vi "Calibration GUI.vi"(7 "Actions":T1, 8 "error in (no error)":errorcluster, 10 "index":i32, 11 "Ctrl Ref":refnum<vi>[](array[refnum])) -> (0 "error out":errorcluster)   [LabVIEW 2011]
uses:
  Controls/typedef_enum_GFV Calibration GUI_actions.ctl
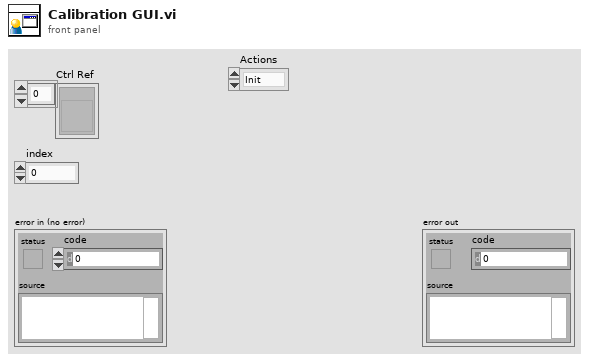
[diagram p1: front panel]
types:
  T1 = typedef "typedef_enum_GFV Calibration GUI_actions.ctl" = enum16{"Init", "Update GUI", "Clear GUI"}
  T2 = enum8{"Enabled", "Disabled", "Disabled and Grayed Out"}
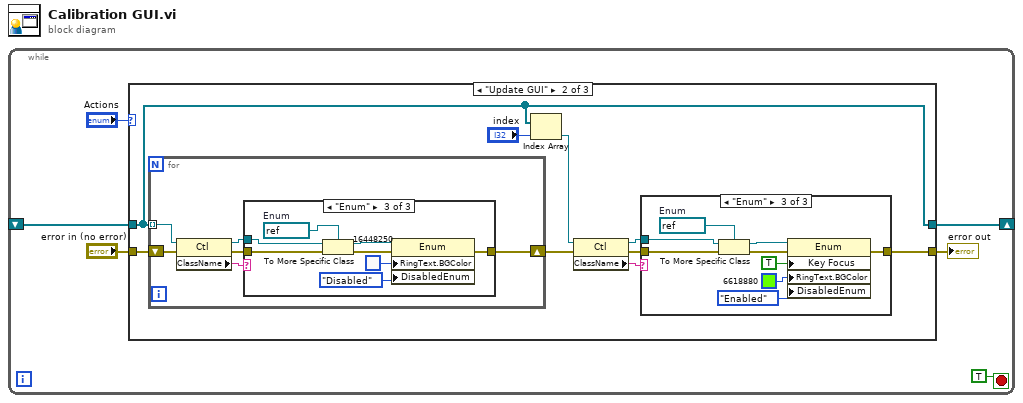
[diagram p0: block diagram]
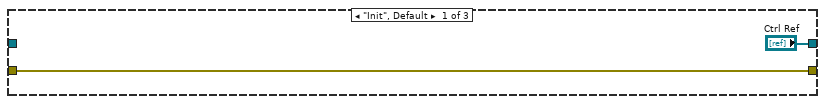
[diagram p2: hidden frame]
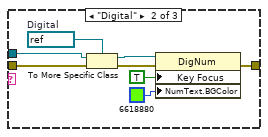
[diagram p4: hidden frame]
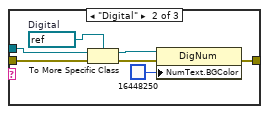
[diagram p6: hidden frame]
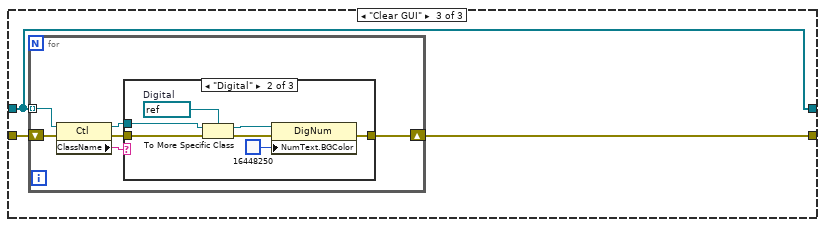
[diagram p7: hidden frame]
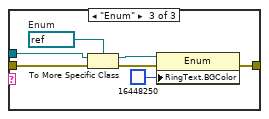
[diagram p9: hidden frame]
diagram:
  n1 = while {
    shift-right: [w2] -> _
    shift-left: _ -> [w1]
    stop <- TRUE stop-if-true
    n2 = case shown="\"Update GUI\"" "Actions" {
      tunnel: [w7 w10 w58] -> w6
      tunnel: "error in (no error)" -> [w7 w17 w60]
      tunnel: ["Ctrl Ref" w15 w59] -> w2
      tunnel: w1 -> [_ w15 w59]
      frame "Init", Default {
      }
      frame "Update GUI" {
        n3 = for {
          tunnel: w15 -> [w41] mode=indexing
          shift-right: [w36] -> w9
          shift-left: w17 -> [w37]
          n4 = property on="Property Node" class="Ctl"(reference=w41, error in=w37) -> (reference out=w39:refnum<vi>, error out=w38:errorcluster, "ClassName"=w40:string)
          n5 = case shown="\"Enum\"" w40 {
            tunnel: w39 -> [_ w47 w55]
            tunnel: w38 -> [w42 w46 w54]
            tunnel: [w42 w45 w53] -> w36
            frame "False", Default {
            }
            frame "Digital" {
              w43 = refnum<vi> refnum  # Digital
              n6 = To More Specific Class(target class=w43, reference=w47, error in=w46) -> (specific class reference=w44:refnum<vi>, error out=w48:errorcluster)
              n7 = property on="Property Node" class="DigNum"(reference=w44, error in=w48, "NumText.BGColor"=u32 16448250) -> (error out=w45:errorcluster)  [unwired: 1 out]
            }
            frame "Enum" {
              w51 = refnum<vi> refnum  # Enum
              n8 = To More Specific Class(target class=w51, reference=w55, error in=w54) -> (specific class reference=w52:refnum<vi>, error out=w56:errorcluster)
              n9 = property on="Property Node" class="Enum"(reference=w52, error in=w56, "RingText.BGColor"=u32 16448250, "DisabledEnum"=T2."Disabled" ("Disabled")) -> (error out=w53:errorcluster)  [unwired: 1 out]
            }
          }
        }
        n10 = Index Array(array=w15, index="index") -> (element=w11:refnum<vi>)
        n11 = property on="Property Node" class="Ctl"(reference=w11, error in=w9) -> (reference out=w13:refnum<vi>, error out=w14:errorcluster, "ClassName"=w12:string)
        n12 = case shown="\"Enum\"" w12 {
          tunnel: w13 -> [_ w25 w34]
          tunnel: w14 -> [w18 w24 w33]
          tunnel: [w18 w23 w32] -> w10
          frame "False", Default {
          }
          frame "Digital" {
            w21 = refnum<vi> refnum  # Digital
            n13 = To More Specific Class(target class=w21, reference=w25, error in=w24) -> (specific class reference=w22:refnum<vi>, error out=w26:errorcluster)
            n14 = property on="Property Node" class="DigNum"(reference=w22, error in=w26, "Key Focus"=TRUE, "NumText.BGColor"=u32 6618880) -> (error out=w23:errorcluster)  [unwired: 1 out]
          }
          frame "Enum" {
            w30 = refnum<vi> refnum  # Enum
            n15 = To More Specific Class(target class=w30, reference=w34, error in=w33) -> (specific class reference=w31:refnum<vi>, error out=w35:errorcluster)
            n16 = property on="Property Node" class="Enum"(reference=w31, error in=w35, "Key Focus"=TRUE, "RingText.BGColor"=u32 6618880, "DisabledEnum"=T2."Enabled" ("Disabled")) -> (error out=w32:errorcluster)  [unwired: 1 out]
          }
        }
      }
      frame "Clear GUI" {
        n17 = for {
          tunnel: w59 -> [w66] mode=indexing
          shift-right: [w61] -> w58
          shift-left: w60 -> [w62]
          n18 = property on="Property Node" class="Ctl"(reference=w66, error in=w62) -> (reference out=w64:refnum<vi>, error out=w63:errorcluster, "ClassName"=w65:string)
          n19 = case shown="\"Digital\"" w65 {
            tunnel: w64 -> [_ w72 w79]
            tunnel: w63 -> [w67 w71 w78]
            tunnel: [w67 w70 w77] -> w61
            frame "False", Default {
            }
            frame "Digital" {
              w68 = refnum<vi> refnum  # Digital
              n20 = To More Specific Class(target class=w68, reference=w72, error in=w71) -> (specific class reference=w69:refnum<vi>, error out=w73:errorcluster)
              n21 = property on="Property Node" class="DigNum"(reference=w69, error in=w73, "NumText.BGColor"=u32 16448250) -> (error out=w70:errorcluster)  [unwired: 1 out]
            }
            frame "Enum" {
              w75 = refnum<vi> refnum  # Enum
              n22 = To More Specific Class(target class=w75, reference=w79, error in=w78) -> (specific class reference=w76:refnum<vi>, error out=w80:errorcluster)
              n23 = property on="Property Node" class="Enum"(reference=w76, error in=w80, "RingText.BGColor"=u32 16448250) -> (error out=w77:errorcluster)  [unwired: 1 out]
            }
          }
        }
      }
    }
    "error out" <- w6
  }
